vi "UI Direct Message.vi"(8 "error in (no error)":errorcluster, 10 "Message Cluster":T1, 11 "Chat Room Model in":refnum<class "Chat Room Model.lvclass">) -> (0 "error out":errorcluster, 3 "Chat Room Model out":refnum<class "Chat Room Model.lvclass">)   [LabVIEW 2020, in "Chat Room Model.lvlib" / "Chat Room Model.lvclass"]
uses:
  Chat Room Model.lvclass
  Chat Room Model.lvclass/Chat Room Model.ctl
  Chat Room Model Messages/Reserve sent message Msg/Reserve sent message Msg.lvclass
  <vilib>/ActorFramework/Actor/Actor.lvclass
  C:/Program Files (x86)/National Instruments/LabVIEW 2020/vi.lib/ActorFramework/Actor/Actor.lvclass
  F:/Gitlab Repository/LabVIEW-Study/10.Top 5 Actor Framework Overrides/Chat Room with Interface/Chat Room Model/Chat Room Model/Chat Room Model.lvclass
  F:/Gitlab Repository/LabVIEW-Study/10.Top 5 Actor Framework Overrides/Chat Room with Interface/Interface/UI Status Change/Chat Room UI.lvclass
  Server/Server Messages/Window Direct Message Msg/Window Direct Message Msg.lvclass
  Application Control/Message.ctl
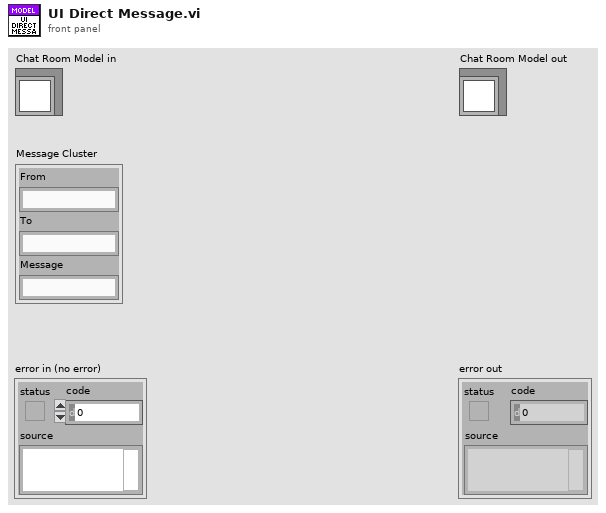
[diagram p1: front panel]
types:
  T1 = typedef "Message.ctl" = cluster{"From":string, "To":string, "Message":string}
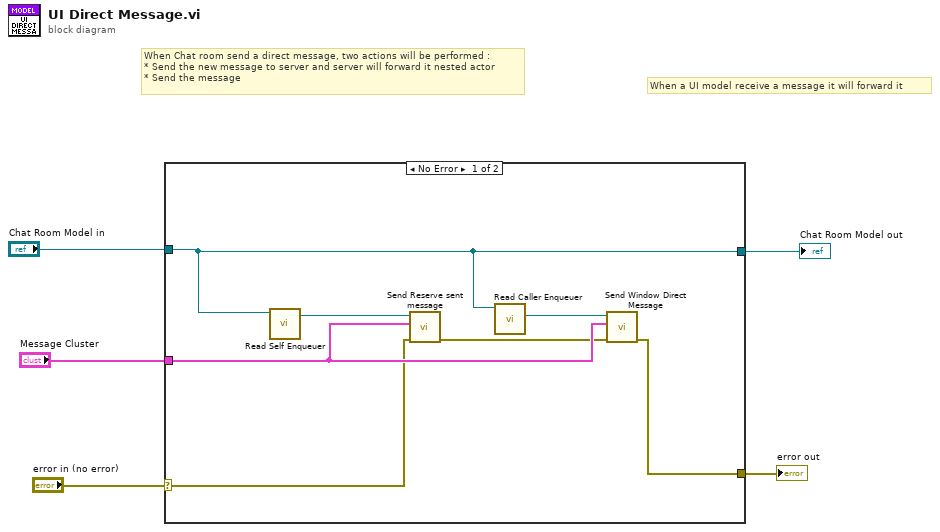
[diagram p0: block diagram]
diagram:
  # "When a UI model receive a message it will forward it"
  # "When Chat room send a direct message, two actions will be performed :\n* Send the new message to server and server will forward it nested actor\n* Send the message"
  n1 = case shown="No Error" "error in (no error)" {
    selector: "error in (no error)" -> [w9 w13]
    tunnel: "Chat Room Model in" -> [w6 w14]
    tunnel: "Message Cluster" -> [w10 _]
    tunnel: [w7 w13] -> w2
    tunnel: [w6 w14] -> w1
    frame No Error {
      n2 = call <vilib>:"Read Self Enqueuer.vi"("Actor"=w6) -> ("Self Enqueuer"=w12:refnum<class "Message Enqueuer.lvclass">)  [unwired: 10 in]
      n3 = call "Send Reserve sent message.vi"("error in (no error)"=w9, "Message Cluster"=w10, "Message Enqueuer"=w12) -> ("error out"=w8:errorcluster)  [unwired: 7 in, 1 out]
      n4 = call <vilib>:"Read Caller Enqueuer.vi"("Actor"=w6) -> ("Caller Enqueuer"=w11:refnum<class "Message Enqueuer.lvclass">)  [unwired: 10 in]
      n5 = call "Send Window Direct Message.vi"("error in (no error)"=w8, "Message Cluster"=w10, "Message Enqueuer"=w11) -> ("error out"=w7:errorcluster)  [unwired: 7 in, 1 out]
    }
    frame Error {
    }
  }
  "error out" <- w2
  "Chat Room Model out" <- w1
